vi "test Can Wait On Multiple Futures.vi"(8 "error in (no error)":errorcluster, 11 "TestCase in":refnum<class "Wait On All Future Tests.lvclass">) -> (0 "error out":errorcluster, 3 "TestCase out":refnum<class "Wait On All Future Tests.lvclass">)   [LabVIEW 2017, in "Wait On All Future Tests.lvclass"]
uses:
  Wait On All Future Tests.lvclass
  <vilib>/addons/_JKI Toolkits/VI Tester/TestCase.llb/TestCase.lvclass
  Futures/Futures.lvlib
  Futures/Promise/Promise.lvclass
  Futures/Future/Future.lvclass
  C:/Program Files (x86)/National Instruments/LabVIEW 2017/vi.lib/addons/_JKI Toolkits/VI Tester/TestCase.llb/TestCase.lvclass
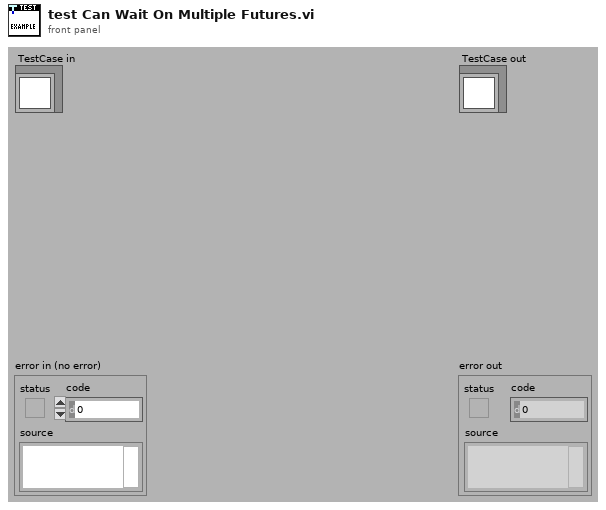
[diagram p1: front panel]
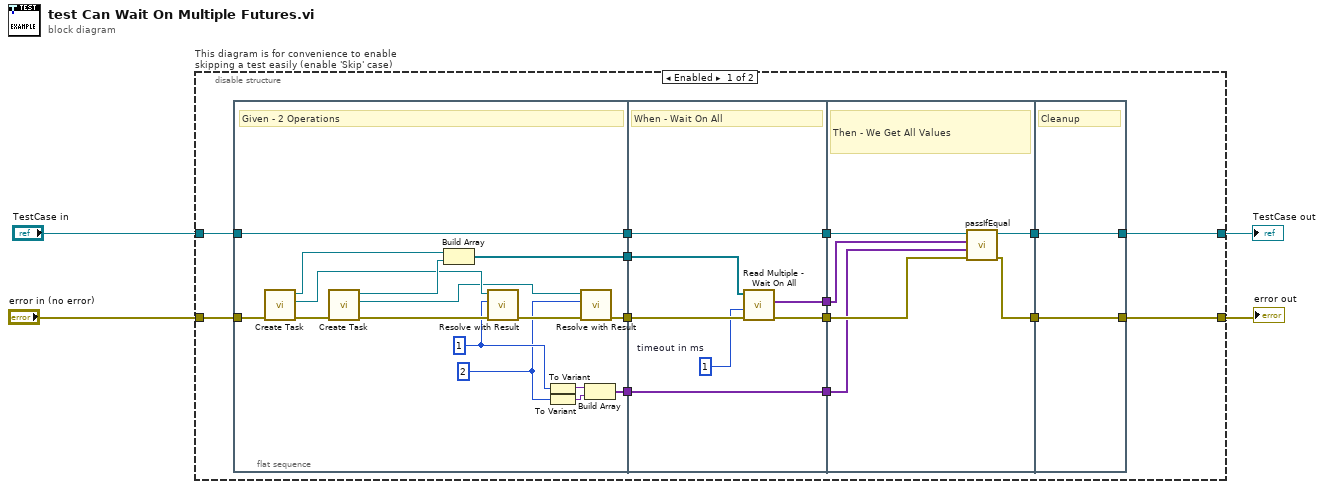
[diagram p0: block diagram]
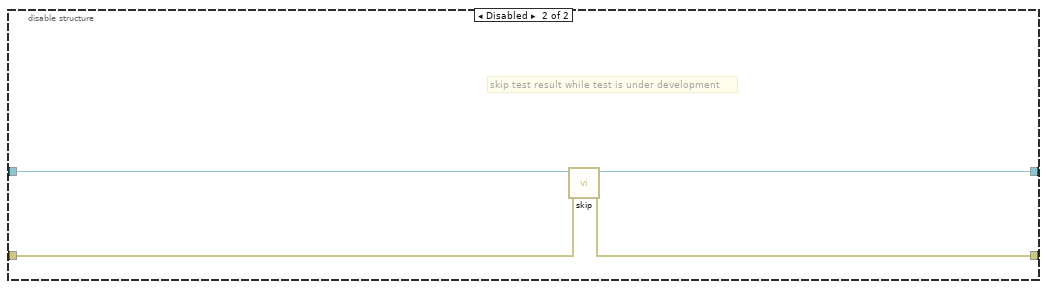
[diagram p2: hidden frame]
diagram:
  n1 = disable-structure "This diagram is for convenience to enable skipping a test easily (enable 'Skip' case)" shown="Enabled" {
    disable-tunnel: "TestCase in" -> [w14 w53]
    disable-tunnel: [w12 w51] -> w1
    disable-tunnel: [w11 w52] -> w3
    disable-tunnel: "error in (no error)" -> [w13 w50]
    frame Enabled {
      n2 = flat-sequence {
        tunnel: w13 -> [w33]
        tunnel: w14 -> [w34]
        tunnel: [w34] -> w18
        tunnel: [w25] -> w9
        tunnel: [w24] -> w8
        tunnel: [w19] -> w5
        tunnel: [w41] -> w17
        tunnel: w18 -> [w41]
        tunnel: [w40] -> w10
        tunnel: w9 -> [w39]
        tunnel: w8 -> [w38]
        tunnel: [w36] -> w7
        tunnel: [w35] -> w6
        tunnel: w5 -> [w35]
        tunnel: [w46] -> w16
        tunnel: [w45] -> w15
        tunnel: w17 -> [w47]
        tunnel: w10 -> [w44]
        tunnel: w7 -> [w43]
        tunnel: w6 -> [w42]
        tunnel: [w48] -> w11
        tunnel: [w49] -> w12
        tunnel: w16 -> [w49]
        tunnel: w15 -> [w48]
        frame #0 {
          w22 = 2
          w23 = 1
          # "Given - 2 Operations"
          n3 = call "Create Task.vi"("error in (no error)"=w33) -> ("error out"=w32:errorcluster, "Promise out"=w27:refnum<class "Promise.lvclass">, "Future out"=w30:refnum<class "Future.lvclass">)  [unwired: 8 in]
          n4 = call "Create Task.vi"("error in (no error)"=w32) -> ("error out"=w29:errorcluster, "Promise out"=w26:refnum<class "Promise.lvclass">, "Future out"=w31:refnum<class "Future.lvclass">)  [unwired: 8 in]
          n5 = Build Array(w30, w31) -> (w25:refnum<class "Future.lvclass">[])
          n6 = call "Resolve with Result.vi"("error in (no error)"=w29, "Result"=w23, "Promise in"=w27) -> ("error out"=w28:errorcluster)  [unwired: 8 in]
          n7 = To Variant(anything=w23) -> (Variant=w21:variant)
          n8 = To Variant(anything=w22) -> (Variant=w20:variant)
          n9 = call "Resolve with Result.vi"("error in (no error)"=w28, "Result"=w22, "Promise in"=w26) -> ("error out"=w24:errorcluster)  [unwired: 8 in]
          n10 = Build Array(w21, w20) -> (w19:variant[])
        }
        frame #1 {
          w37 = 1  # timeout in ms
          # "When - Wait On All"
          n11 = call "Read Multiple - Wait On All.vi"("error in (no error)"=w38, "timeout in ms (60 sec)"=w37, "Futures in"=w39) -> ("error out"=w40:errorcluster, "Result value"=w36:variant[])  [unwired: 5 in, 2 out]
        }
        frame #2 {
          # "Then - We Get All Values"
          n12 = call-dynamic "passIfEqual.vi"("error in (no error)"=w44, "y"=w42, "x"=w43, "TestCase in"=w47) -> ("error out"=w45:errorcluster, "TestCase out"=w46:refnum<class "Wait On All Future Tests.lvclass">)  [unwired: 6 in]
        }
        frame #3 {
          # "Cleanup"
        }
      }
    }
    frame Disabled {
      # "skip test result while test is under development"
      n13 = call <vilib>:"skip.vi"("error in (no error)"=w50, "TestCase in"=w53) -> ("error out"=w52:errorcluster, "TestCase out"=w51:refnum<class "Wait On All Future Tests.lvclass">)  [unwired: 8 in]
    }
  }
  "error out" <- w3
  "TestCase out" <- w1
